vi "Stop Core.vi"(10 "final error code":i32, 11 "Hamamatsu_Camera in":refnum<class "Hamamatsu_Camera.lvclass">) -> (3 "Hamamatsu_Camera out":refnum<class "Hamamatsu_Camera.lvclass">)   [LabVIEW 2023, in "Hamamatsu_Camera.lvlib" / "Hamamatsu_Camera.lvclass"]
doc: "(<B>Filename</B>: Actor Framework.lvlib:Actor.lvclass:Stop Core.vi)\n\nDefines what the actor does before it stops. Use the <B>final error code</B> input to determine whether the actor shut down in response to an error.\n\nBy default, this method passes the Stop message along to all auto-stop nested actors. A descendant class may override this method to define additional behavior, such as shutting down any processes the actor initiated in its override of the Actor Core method."
uses:
  Hamamatsu_Camera.lvclass
  Hamamatsu_Camera.lvclass/Hamamatsu_Camera.ctl
  <vilib>/ActorFramework/Actor/Actor.lvclass
panel:
  out "Capturing":bool=TRUE
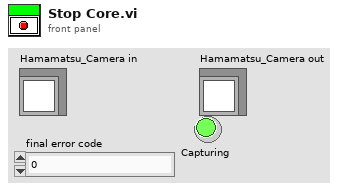
[diagram p1: front panel]
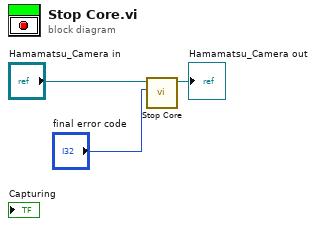
[diagram p0: block diagram]
diagram:
  n1 = call-parent "Stop Core.vi"("final error code"="final error code", "Actor in"="Hamamatsu_Camera in") -> ("Actor out"=→"Hamamatsu_Camera out":refnum<class "Hamamatsu_Camera.lvclass">)  [unwired: 9 in]
